vi "Router - Data Integrity - Organized.vi"() -> ()   [LabVIEW 2016]
uses:
  XML Cluster.ctl
  Node Properties.ctl
  <vilib>/Utility/error.llb/DialogType.ctl
  <vilib>/Platform/TimedLoop/XDataNode/timing_clust.ctl
  <vilib>/Platform/TimedLoop/XDataNode/nitl_modes.ctl
  <vilib>/Platform/TimedLoop/XDataNode/wakeup.ctl
  <vilib>/pximc/Initialize Writer Session (DBL).vi
  <vilib>/pximc/Connect (DBL).vi
  <vilib>/pximc/Initialize Reader Session (DBL).vi
  <vilib>/pximc/Acquire Read Region (DBL).vi
  <vilib>/pximc/Acquire Write Region (DBL).vi
  <vilib>/platform/TimedLoop/XDataNode/XDataNode.xnode
  <vilib>/pximc/nipximc.lvlib
  <resource>/objmgr/pximc.rc
  <vilib>/Platform/TimedLoop/XDataNode/XDNodeRunTimeDep.lvlib
panel:
  in  "Configuration Properties":T1={"Node Properties"=[{"Resource Name"="PXI1Slot2", "Slave IP Address"="", "Node ID"=1, "Node # Channels"=2, "Data Importing Nodes"=[]}, {"Resource Name"="PXI1Slot2", "Slave IP Address"="", "Node ID"=2, "Node # Channels"=2, "Data Importing Nodes"=[]}], "Connection Timeout (s)"=60.0, "Readers Buffer Size"=250000}
  out "Waveform Chart 3":T3(graph)={"[0]"=0.45399049973957295, "[1]"=-0.809016994374982, "[2]"=0.9876883405951427, "[3]"=0.7071067811864036, "[4]"=1.0, "[5]"=0.7071067811869794, "[6]"=0.0, "[7]"=0.0, "[8]"=0.0}
  in  "Stop Button":bool
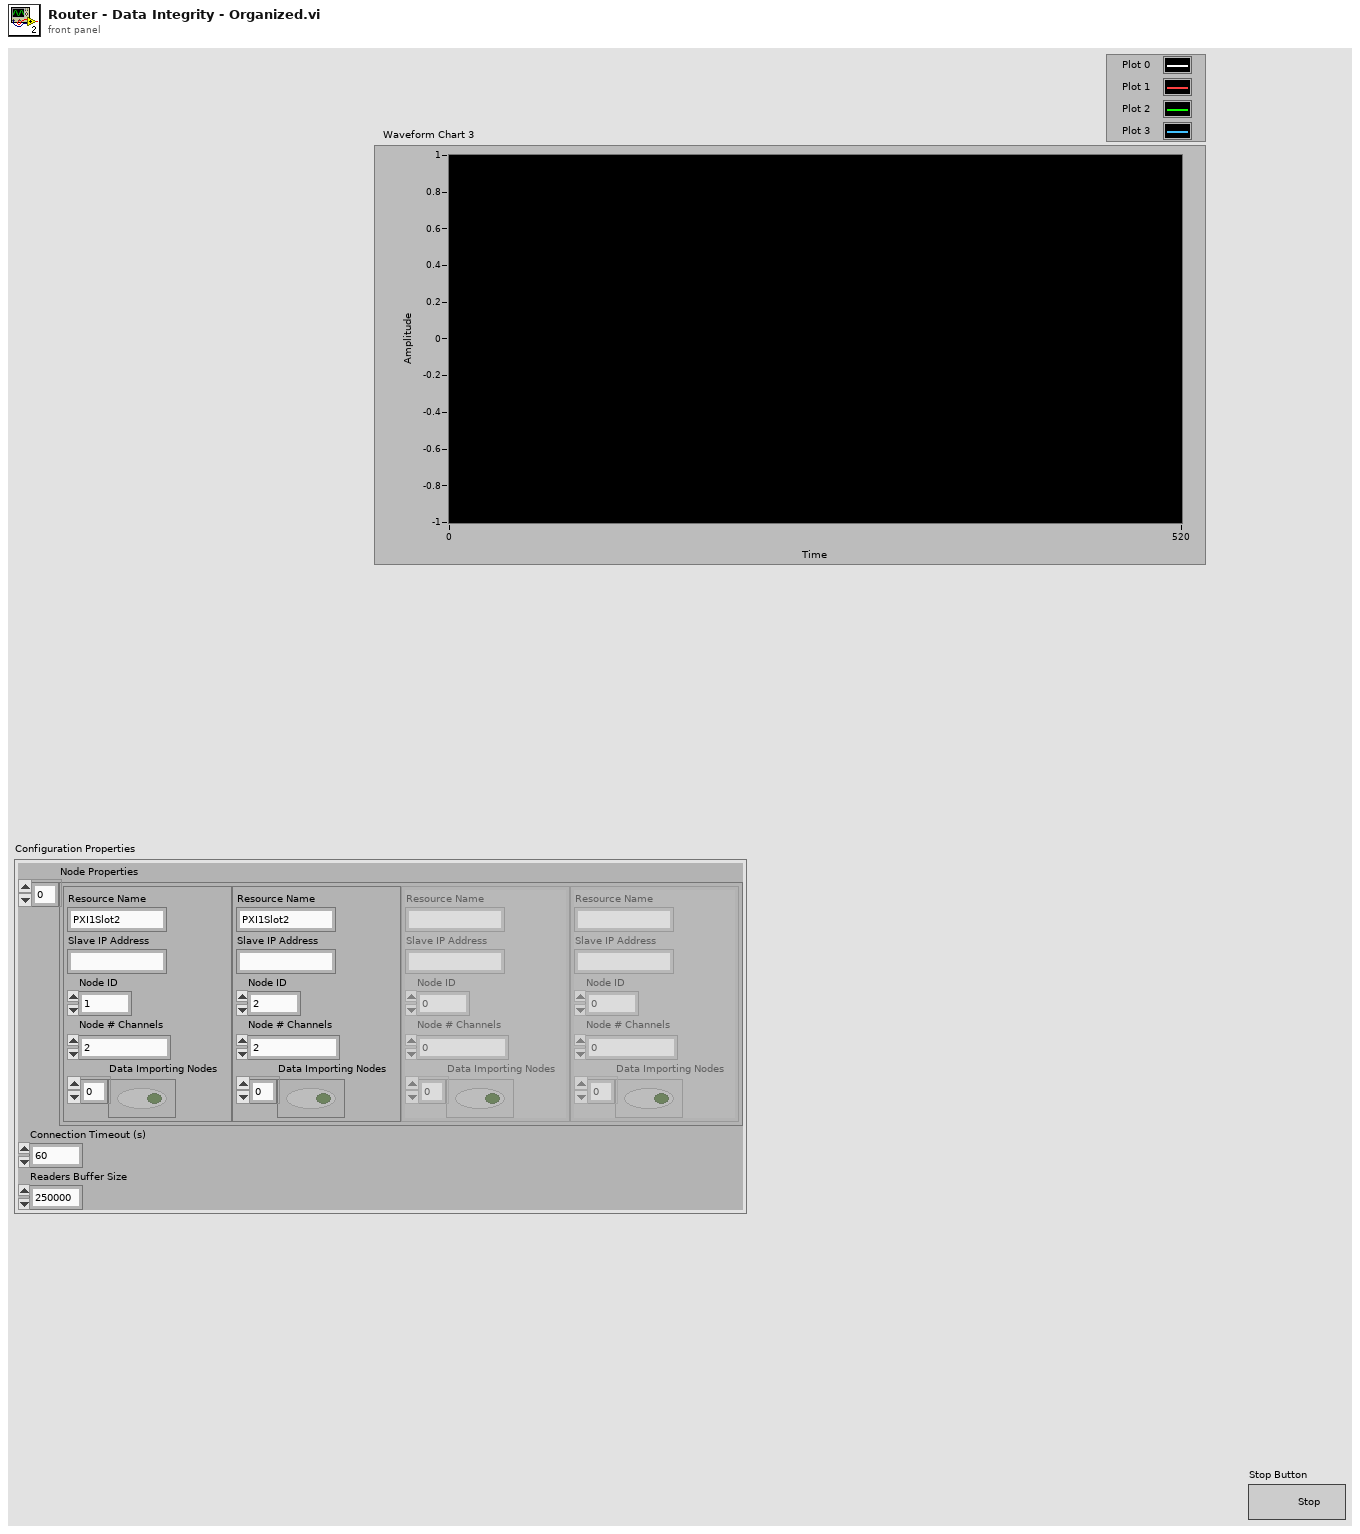
[diagram p1: front panel]
types:
  T1 = typedef "XML Cluster.ctl" = cluster{"Node Properties":T2[], "Connection Timeout (s)":dbl, "Readers Buffer Size":u32}
  T2 = typedef "Node Properties.ctl" = cluster{"Resource Name":string, "Slave IP Address":string, "Node ID":u16, "Node # Channels":u32, "Data Importing Nodes":bool[]}
  T3 = cluster{"[0]":dbl, "[1]":dbl, "[2]":dbl, "[3]":dbl, "[4]":dbl, "[5]":dbl, "[6]":dbl, "[7]":dbl, "[8]":dbl}
  T4 = typedef "DialogType.ctl" = u16
  T5 = typedef "XDNodeRunTimeDep.lvlib/timing_clust.ctl" = cluster{"Expected End [f-1]":u64, "Actual End [f-1]":u64, "Finished Late? [f-1]":bool, "Expected End [i-1]":u64, "Actual End [i-1]":u64, "Finished Late? [i-1]":bool, "Expected Start [i]":u64, "Actual Start [i]":u64, "Expected Start [f]":u64, "Actual Start [f]":u64, "Source Name":string, "Structure Name":string, "Period":i64, "Deadline":i64, "Offset":i64, "Start":i64, "Priority":i32, "Timeout":i32, "Mode":T6, "Wakeup Reason":T7, "Error":errorcluster, "Source Type":string, "Secondary Source Type":string, "Global End Time":u64, "Global Start Time":u64, "Frame Duration":u64, "Iteration Duration":u64, "Assigned CPU":i32, "I/O Scan Engine Mode":u32}
  T6 = typedef "XDNodeRunTimeDep.lvlib/nitl_modes.ctl" = enum32{"No Change", "Process missed periods, maintain original phase", "Discard missed periods, maintain original phase", "Process missed periods, ignore original phase", "Discard missed periods, ignore original phase"}
  T7 = typedef "XDNodeRunTimeDep.lvlib/wakeup.ctl" = enum32{"Normal", "Aborted", "Asynchronous wakeup", "Timing source error", "Timed loop error", "Timeout"}
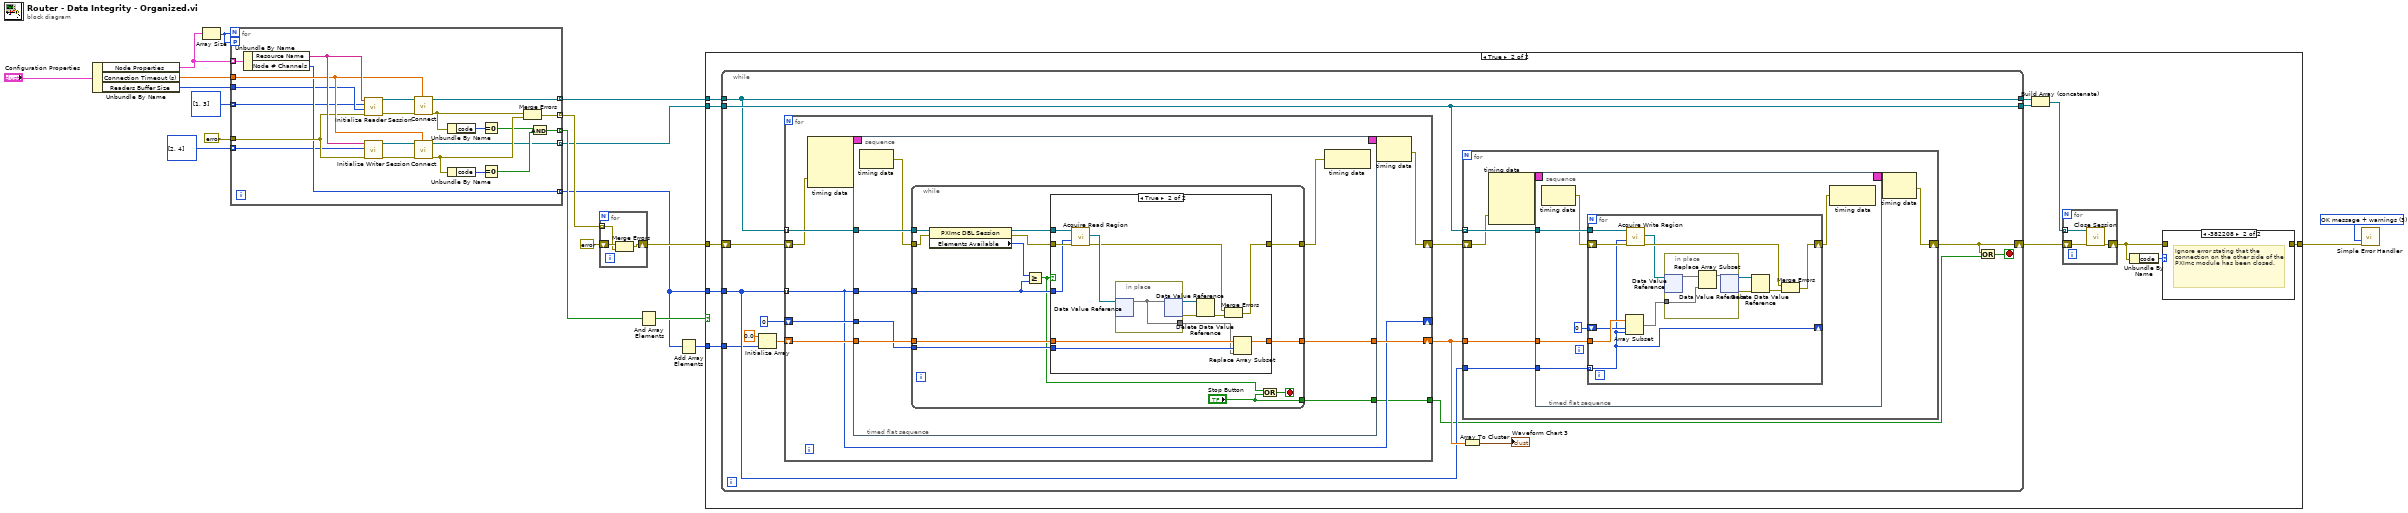
[diagram p0: block diagram]
diagram:
  w4 = T4 3 items=["no dialog", "OK message", "continue or stop message", "OK message + warnings", "continue/stop + warnings"] ("type of dialog (OK msg:1)")
  n1 = Unbundle By Name("Configuration Properties") -> ("Node Properties"=w18:T2[], "Connection Timeout (s)"=w16:dbl, "Readers Buffer Size"=w3:u32)
  n2 = Array Size(array=w18) -> (size(s)=w17:i32)
  n3 = for {
    N: w17 -> [_]
    tunnel: w18 -> [w41] mode=indexing
    workers-P: w17 -> [_]
    tunnel: w16 -> [w37]
    tunnel: errorcluster {"status"=FALSE, "code"=0, "source"=""} ("error constant") -> [w35]
    tunnel: [w27] -> w14 mode=indexing
    tunnel: [w26] -> w8 mode=indexing
    tunnel: [w25] -> w9 mode=indexing
    tunnel: [w24] -> w6 mode=indexing
    tunnel: [w23] -> w11 mode=indexing
    tunnel: w3 -> [w22]
    tunnel: i32[] [2, 4] -> [w21] mode=indexing
    tunnel: i32[] [1, 3] -> [w20] mode=indexing
    n4 = Unbundle By Name(w41) -> ("Resource Name"=w40:string, "Node # Channels"=w24:u32)
    n5 = call-poly <vilib>:"Initialize Reader Session.vi"("error in (no error)"=w35, "buffer size"=w22, "writer's connection id (1)"=w20, "interface"=w40) -> ("error out"=w38:errorcluster, "session out"=w39:refnum<k21>)  [unwired: 6 in]
    n6 = call-poly <vilib>:"Initialize Writer Session.vi"("error in (no error)"=w35, "connection id (1)"=w21, "interface"=w40) -> ("error out"=w36:errorcluster, "session out"=w32:refnum<k21>)  [unwired: 7 in]
    n7 = call-poly <vilib>:"Connect.vi"("timeout in seconds (-1)"=w37, "error in (no error)"=w38, "session in"=w39) -> ("error out"=w33:errorcluster, "session out"=w25:refnum<k21>)  [unwired: 7 in]
    n8 = call-poly <vilib>:"Connect.vi"("timeout in seconds (-1)"=w37, "error in (no error)"=w36, "session in"=w32) -> ("error out"=w30:errorcluster, "session out"=w26:refnum<k21>)  [unwired: 7 in]
    n9 = Unbundle By Name(w33) -> ("code"=w34:i32)
    n10 = Unbundle By Name(w30) -> ("code"=w31:i32)
    n11 = Equal To 0?(x=w34) -> (x = 0?=w29:bool)
    n12 = Equal To 0?(x=w31) -> (x = 0?=w28:bool)
    n13 = Merge Errors(w33, w30) -> (w23:errorcluster)
    n14 = And(x=w29, y=w28) -> (x .and. y?=w27:bool)
  }
  n15 = for {
    tunnel: w11 -> [w43] mode=indexing
    shift-right: [w42] -> w7
    shift-left: errorcluster {"status"=FALSE, "code"=0, "source"=""} ("error constant") -> [w44]
    n16 = Merge Errors(w44, w43) -> (w42:errorcluster)
  }
  n17 = And Array Elements(Boolean array=w14) -> (logical AND=w12:bool)
  n18 = Add Array Elements(numeric array=w6) -> (sum=w13:u32)
  n19 = case shown="True" w12 {
    tunnel: w9 -> [_ w57]
    tunnel: w8 -> [_ w56]
    tunnel: [w45 w49] -> w5
    tunnel: w7 -> [w45 w48]
    tunnel: w6 -> [_ w47]
    tunnel: w13 -> [_ w46]
    frame False {
    }
    frame True {
      n20 = while {
        tunnel: w57 -> [w63]
        tunnel: w56 -> [w68]
        shift-right: [w70] -> w54
        shift-left: w48 -> [w69]
        tunnel: [w63] -> w53
        tunnel: [w68] -> w52
        tunnel: w47 -> [w62]
        tunnel: w46 -> [w61]
        stop <- w58 stop-if-true
        n21 = Initialize Array(0.0 ("element"), w61) -> (w66:dbl[])
        n22 = for {
          shift-right: [w73] -> w71
          shift-left: w69 -> [w72]
          tunnel: w63 -> [w81] mode=indexing
          shift-right: [w79] -> w64
          shift-left: w66 -> [w80]
          tunnel: w62 -> [w77] mode=indexing
          shift-right: [w77] -> _
          shift-left: u64 0 ("y") -> [w78]
          tunnel: [w76] -> w59
          n23 = node-c288(w72) -> (w75:T5)  [unwired: 3 in]
          n24 = timed-sequence {
            timing: w75 -> [_]
            timing-out: [_] -> w74
            tunnel: w81 -> [w87]
            tunnel: w80 -> [w86]
            tunnel: [w85] -> w79
            tunnel: w78 -> [w84]
            tunnel: w77 -> [w83]
            tunnel: [w82] -> w76
            n25 = timed-flat-sequence {
              tunnel: w87 -> [w95]
              tunnel: w86 -> [w94]
              tunnel: [w93] -> w85
              tunnel: w84 -> [w92]
              tunnel: w83 -> [w91]
              tunnel: [w90] -> w82
              n26 = node-c288() -> (w88:errorcluster)  [unwired: 1 in]
              n27 = while {
                tunnel: w95 -> [w107]
                tunnel: w88 -> [w104]
                tunnel: [w108] -> w89
                tunnel: w94 -> [w102]
                tunnel: [w101] -> w93
                tunnel: w91 -> [w100]
                tunnel: w92 -> [w99]
                tunnel: ["Stop Button"] -> w90
                stop <- w97 stop-if-true
                n28 = property class="PXImc DBL Session"(reference=w107, error in=w104) -> (reference out=w105:refnum<k21>, error out=w103:errorcluster, "Elements Available"=w106:u64)
                n29 = Greater Or Equal?(x=w106, y=w100) -> (x >= y?=w98:bool)
                n30 = case shown="True" w98 {
                  tunnel: w103 -> [w110 w122]
                  tunnel: [w110 w116] -> w108
                  tunnel: w105 -> [_ w121]
                  tunnel: w102 -> [w109 w115]
                  tunnel: w99 -> [_ w114]
                  tunnel: [w109 w112] -> w101
                  tunnel: w100 -> [_ w111]
                  frame False {
                  }
                  frame True {
                    n31 = call-poly <vilib>:"Acquire Read Region.vi"("error in (no error)"=w122, "number of elements"=w111, "session in"=w121) -> ("error out"=w117:errorcluster, "read region reference"=w123:refnum<data-value>)  [unwired: 5 in, 2 out]
                    n32 = in-place {
                      in-place-border: [w124] -> w113
                      n33 = in-place-dvr #1(w123) -> (w124:dbl[])  [unwired: 1 out]
                      n34 = in-place-dvr #1(w124) -> (w120:refnum<data-value>, w119:errorcluster)
                    }
                    n35 = Delete Data Value Reference(data value reference=w120, error in=w119) -> (error out=w118:errorcluster)  [unwired: 1 out]
                    n36 = Merge Errors(w117, w118) -> (w116:errorcluster)
                    n37 = Replace Array Subset(array=w115, new element=w113, index=w114) -> (w112:dbl[])
                  }
                }
                n38 = Or(x=w98, y="Stop Button") -> (x .or. y?=w97:bool)
              }
              n39 = node-c288(w89) -> ()  [unwired: 1 out]
            }
          }
          n40 = node-c288(w74) -> (w73:errorcluster)
        }
        n41 = for {
          tunnel: w68 -> [w141] mode=indexing
          tunnel: w64 -> [w140]
          tunnel: w62 -> [w139]
          shift-right: [w136] -> w70
          shift-left: w71 -> [w135]
          n42 = node-c288(w135) -> (w138:T5)  [unwired: 3 in]
          n43 = timed-sequence {
            timing: w138 -> [_]
            timing-out: [_] -> w137
            tunnel: w141 -> [w144]
            tunnel: w140 -> [w143]
            tunnel: w139 -> [w142]
            n44 = timed-flat-sequence {
              tunnel: w144 -> [w150]
              tunnel: w143 -> [w149]
              tunnel: w142 -> [w148]
              n45 = node-c288() -> (w146:errorcluster)  [unwired: 1 in]
              n46 = for {
                tunnel: w150 -> [w162]
                shift-right: [w160] -> w145
                shift-left: w146 -> [w161]
                tunnel: w149 -> [w157]
                tunnel: w148 -> [w151] mode=indexing
                shift-right: [w151] -> _
                shift-left: u64 0 ("y") -> [w152]
                n47 = Array Subset(array=w157, index=w152, length=w151) -> (w156:dbl[])
                n48 = call-poly <vilib>:"Acquire Write Region.vi"("error in (no error)"=w161, "number of elements"=w151, "session in"=w162) -> ("error out"=w159:errorcluster, "write region reference"=w158:refnum<data-value>)  [unwired: 5 in, 2 out]
                n49 = in-place {
                  in-place-border: w156 -> [w163]
                  n50 = in-place-dvr #2(w158) -> (w165:dbl[])  [unwired: 1 out]
                  n51 = Replace Array Subset(array=w165, new element=w163) -> (w164:dbl[])  [unwired: 1 in]
                  n52 = in-place-dvr #2(w164) -> (w155:refnum<data-value>, w153:errorcluster)
                }
                n53 = Delete Data Value Reference(data value reference=w155, error in=w153) -> (error out=w154:errorcluster)  [unwired: 1 out]
                n54 = Merge Errors(w159, w154) -> (w160:errorcluster)
              }
              n55 = node-c288(w145) -> ()  [unwired: 1 out]
            }
          }
          n56 = node-c288(w137) -> (w136:errorcluster)
        }
        n57 = Array To Cluster(array=w64) -> (cluster=→"Waveform Chart 3":T3)
        n58 = Or(x=w70, y=w59) -> (x .or. y?=w58:bool)
      }
      n59 = Build Array (concatenate)(w53, w52) -> (w51:refnum<k21>[])
      n60 = for {
        tunnel: w51 -> [w178] mode=indexing
        shift-right: [w176] -> w50
        shift-left: w54 -> [w177]
        n61 = call <vilib>:"Close Session.vi"("error in (no error)"=w177, "session in"=w178) -> ("error out"=w176:errorcluster)  [unwired: 9 in]
      }
      n62 = Unbundle By Name(w50) -> ("code"=w55:i32)
      n63 = case shown="-382208" w55 {
        tunnel: w50 -> [w179 _]
        tunnel: [w179 _] -> w49
        frame 0, Default {
        }
        frame -382208 {
          # "Ignore error stating that the connection on the other side of the PXImc module has been closed."
        }
      }
    }
  }
  n64 = call <vilib>:"Simple Error Handler.vi"("type of dialog (OK msg:1)"=w4, "error in (no error)"=w5) -> ()  [unwired: 3 in, 5 out]
